vi "DIFFERENT TYPES OF COMPARISION OPERATORS 1.vi"() -> ()   [LabVIEW 2019]
panel:
  out "OUTPUT FOR EQUAL TO":bool
  out "OUTPUT FOR LESS THAN OR EQUAL TO":bool
  out "OUTPUT FOR GREATER THAN OR EQUAL TO":bool
  out "OUTPUT FOR LESS THAN":bool
  out "OUTPUT FOR GREATER THAN":bool
  out "OUTPUT FOR NOT EQUAL TO":bool
  in  "INPUT 2":dbl
  in  "INPUT 1":dbl
  # "DIFFERENT TYPES OF COMPARISION OPERATORS-1"
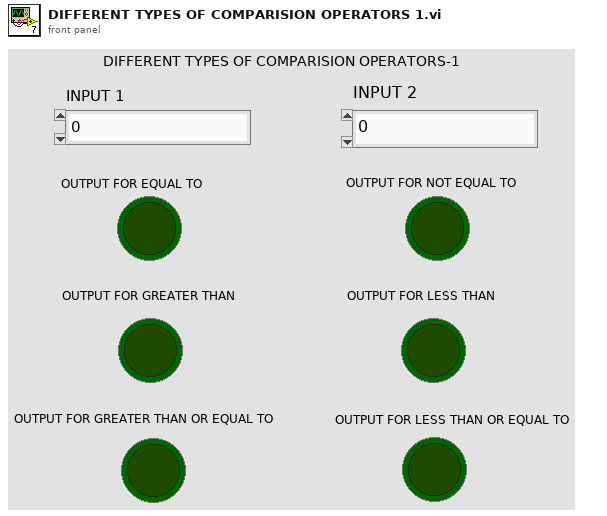
[diagram p1: front panel]
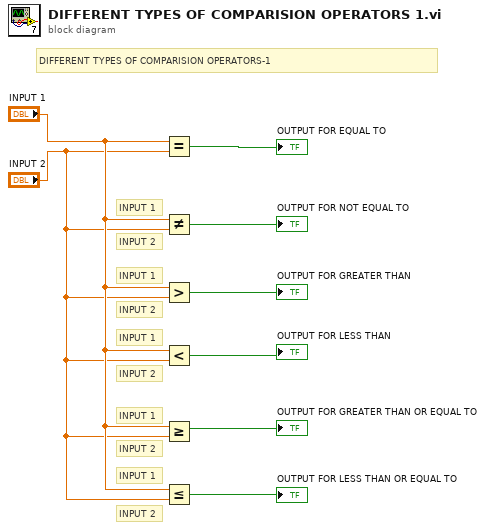
[diagram p0: block diagram]
diagram:
  # "INPUT 2"
  # "INPUT 2"
  # "INPUT 2"
  # "INPUT 2"
  # "INPUT 2"
  # "INPUT 1"
  # "INPUT 1"
  # "INPUT 1"
  # "INPUT 1"
  # "INPUT 1"
  # "DIFFERENT TYPES OF COMPARISION OPERATORS-1"
  n1 = Equal?(x="INPUT 1", y="INPUT 2") -> (x = y?=→"OUTPUT FOR EQUAL TO":bool)
  n2 = Not Equal?(x="INPUT 1", y="INPUT 2") -> (x != y?=→"OUTPUT FOR NOT EQUAL TO":bool)
  n3 = Greater?(x="INPUT 1", y="INPUT 2") -> (0:→"OUTPUT FOR GREATER THAN":bool)
  n4 = Less?(x="INPUT 1", y="INPUT 2") -> (x < y?=→"OUTPUT FOR LESS THAN":bool)
  n5 = Greater Or Equal?(x="INPUT 1", y="INPUT 2") -> (x >= y?=→"OUTPUT FOR GREATER THAN OR EQUAL TO":bool)
  n6 = Less Or Equal?(x="INPUT 1", y="INPUT 2") -> (x <= y?=→"OUTPUT FOR LESS THAN OR EQUAL TO":bool)
